vi "config.vi"(0 "System locator":string(combo)="usb:id:425839965", 1 "X channel":u32=1, 2 "Y channel":u32=2, 3 "Rotation channel":u32, 4 "error in (no error)":errorcluster) -> (5 "error out":errorcluster)   [LabVIEW 2016]
uses:
  sa commands.ctl
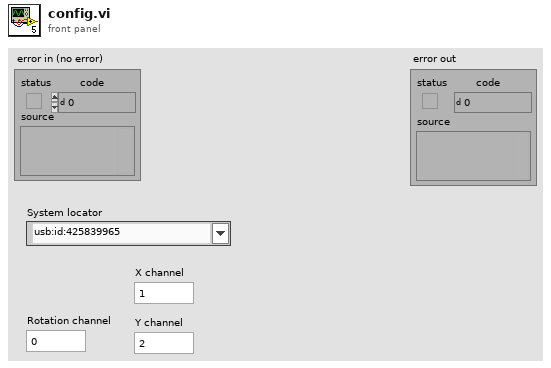
[diagram p1: front panel]
types:
  T1 = typedef "sa commands.ctl" = enum16{"read all", "set system index", "set x channel", "set y channel", "set rotation channel"}
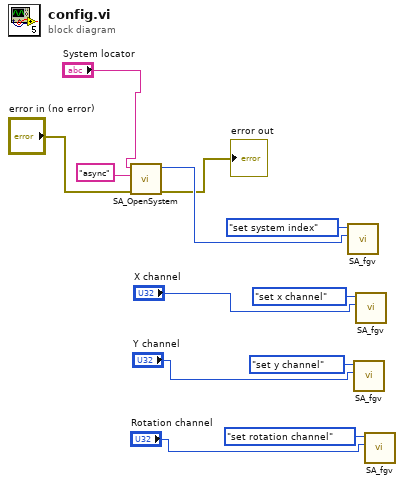
[diagram p0: block diagram]
diagram:
  n1 = call <vilib>:"SA_OpenSystem.vi"("error in (no error)"="error in (no error)", "options"="async", "systemLocator"="System locator") -> ("error out"=→"error out":errorcluster, "systemIndexOut"=w4:u32)  [unwired: 7 in]
  n2 = call "SA_fgv.vi"("value"=w4, "command"=sa_commands."set system index") -> ()  [unwired: 2 in, 4 out]
  n3 = call "SA_fgv.vi"("value"="Y channel", "command"=sa_commands."set y channel") -> ()  [unwired: 2 in, 4 out]
  n4 = call "SA_fgv.vi"("value"="X channel", "command"=sa_commands."set x channel") -> ()  [unwired: 2 in, 4 out]
  n5 = call "SA_fgv.vi"("value"="Rotation channel", "command"=sa_commands."set rotation channel") -> ()  [unwired: 2 in, 4 out]
